vi "4155C Output-FPP Config SMUs v3.0.vi"(0 "VISA resource name in":refnum<visa-resource-name>, 1 "Pulse period":dbl=0.005 min=0.005 max=1.0 step=0.0001 format="%.4f", 2 "FPP - Source":u32(ring)=6 items=["SMU1  ", "SMU2  ", "SMU3  ", "SMU4  ", "SMU5  ", "SMU6  ", "VSU1  ", "VSU2  "], 3 "Pulse width":dbl=0.0005 min=0.0005 max=0.1 step=0.0001 format="%.4f", 4 "Base voltage":dbl format="%^.4e", 5 "error in (no error)":errorcluster, 6 "sweep method":u16(ring) items=["Continuous", "Pulsed"], 7 "FPP - Gate":u32(ring)=2 items=["SMU1  ", "SMU2  ", "SMU3  ", "SMU4  ", "SMU5  ", "SMU6  ", "VSU1  ", "VSU2  "], 8 "FPP - Drain":u32(ring)=1 items=["SMU1  ", "SMU2  ", "SMU3  ", "SMU4  ", "SMU5  ", "SMU6  ", "VSU1  ", "VSU2  "], 9 "FPP - Probe 1":u32(ring) items=["SMU1  ", "SMU2  ", "SMU3  ", "SMU4  ", "SMU5  ", "SMU6  ", "VSU1  ", "VSU2  "], 10 "Gate mode":u16(ring) items=["Auto", "Limited", "Fixed"], 11 "Source/drain mode":u16(ring) items=["Auto", "Limited", "Fixed"], 12 "Gate Range":u8(slide)=6 max=11 scale=0.0..11.0, 13 "Source/drain Range":u8(slide)=6 max=11 scale=0.0..11.0, 15 "FPP - Probe 2":u32(ring)=3 items=["SMU1  ", "SMU2  ", "SMU3  ", "SMU4  ", "SMU5  ", "SMU6  ", "VSU1  ", "VSU2  "]) -> (14 "VISA Resource Name out":refnum<visa-resource-name>, 19 "error out":errorcluster)   [LabVIEW 2016]
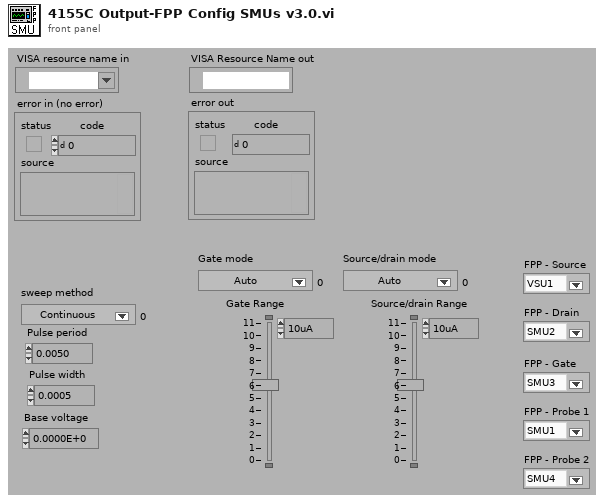
[diagram p1: front panel]
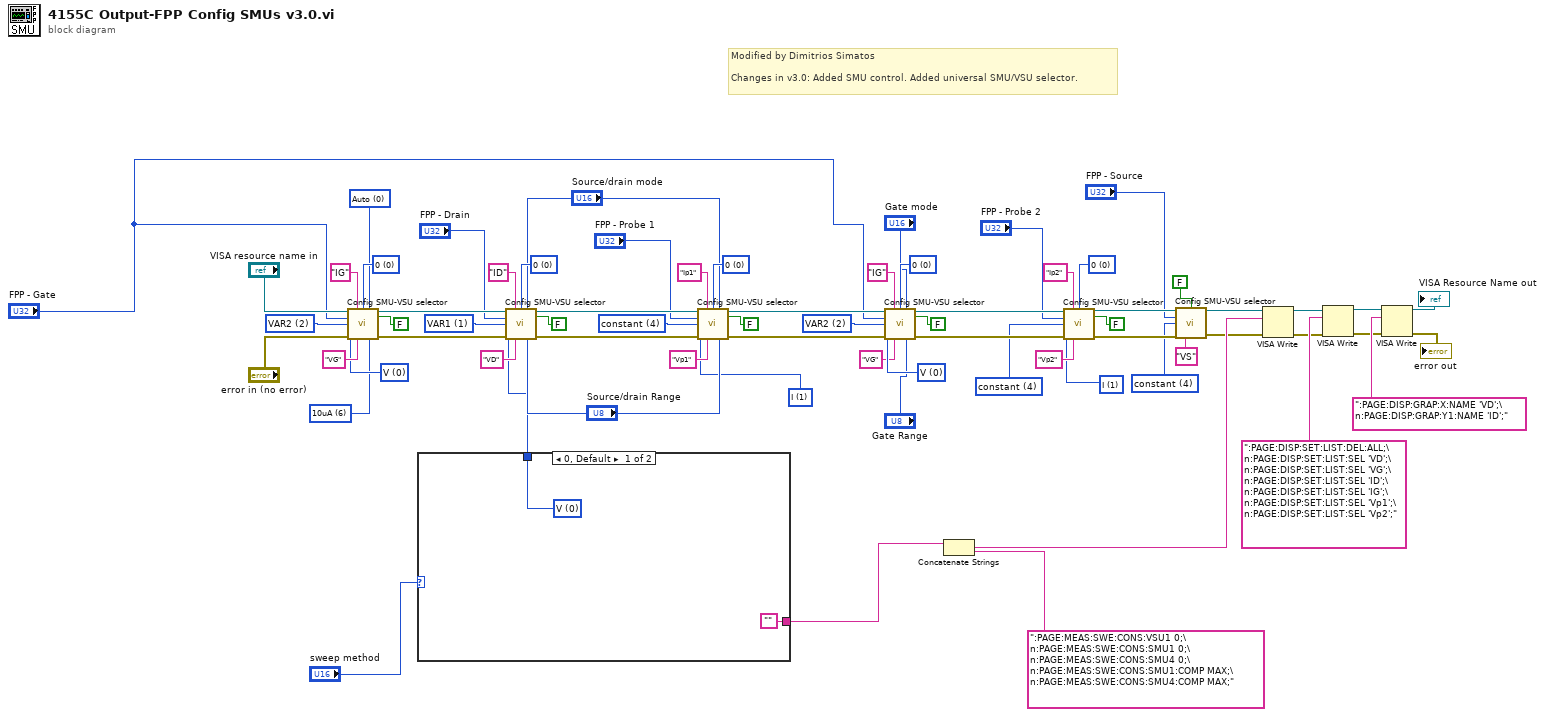
[diagram p0: block diagram]
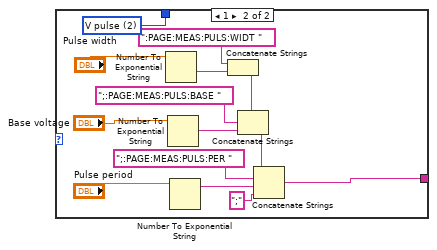
[diagram p2: hidden frame]
diagram:
  w19 = u32 4 items=["disabled  ", "VAR1  ", "VAR2  ", "VAR1'  ", "constant  "] ("function")
  w23 = u32 4 items=["disabled  ", "VAR1  ", "VAR2  ", "VAR1'  ", "constant  "] ("function")
  w25 = u32 1 items=["V  ", "I  ", "V pulse  ", "I pulse  ", "  common  "] ("mode")
  w26 = u16 0 items=["Auto", "Limited", "Fixed"] ("Range mode")
  w27 = u8 6 items=["10fA  ", "100fA  ", "1nA  ", "10nA", "100nA", "1uA", "10uA", "100uA", "1mA", "10mA", "100mA", "1A"] ("Range")
  w32 = u32 2 items=["disabled  ", "VAR1  ", "VAR2  ", "VAR1'  ", "constant  "] ("function")
  w34 = u32 0 items=["0  ", "10K Ohms  ", "100K Ohms  ", "1M Ohms  "] ("series resistance *")
  w35 = u32 0 items=["V  ", "I  ", "V pulse  ", "I pulse  ", "  common  "] ("mode")
  w53 = u32 0 items=["0  ", "10K Ohms  ", "100K Ohms  ", "1M Ohms  "] ("series resistance *")
  w57 = u32 0 items=["V  ", "I  ", "V pulse  ", "I pulse  ", "  common  "] ("mode")
  w58 = u32 0 items=["0  ", "10K Ohms  ", "100K Ohms  ", "1M Ohms  "] ("series resistance *")
  w60 = u32 2 items=["disabled  ", "VAR1  ", "VAR2  ", "VAR1'  ", "constant  "] ("function")
  w63 = u32 0 items=["0  ", "10K Ohms  ", "100K Ohms  ", "1M Ohms  "] ("series resistance *")
  w65 = u32 4 items=["disabled  ", "VAR1  ", "VAR2  ", "VAR1'  ", "constant  "] ("function")
  w39 = u32 1 items=["V  ", "I  ", "V pulse  ", "I pulse  ", "  common  "] ("mode")
  w68 = u32 0 items=["0  ", "10K Ohms  ", "100K Ohms  ", "1M Ohms  "] ("series resistance *")
  w70 = u32 1 items=["disabled  ", "VAR1  ", "VAR2  ", "VAR1'  ", "constant  "] ("function")
  # "Modified by Dimitrios Simatos\n\nChanges in v3.0: Added SMU control. Added universal SMU/VSU selector."
  n1 = call "Config SMU-VSU selector.vi"("VISA session"="VISA resource name in", "I name (max 6 chars)"="IG", "standby"=FALSE, "Range mode"=w26, "unit to configure"="FPP - Gate", "function"=w32, "mode"=w35, "error in (no error)"="error in (no error)", "V name (max 6 chars)"="VG", "series resistance *"=w34, "Range"=w27) -> ("dup VISA resource name"=w29:refnum<visa-resource-name>, "error out"=w30:errorcluster)  [unwired: 1 in, 2 out]
  n2 = case shown="0, Default" "sweep method" {
    tunnel: [w72 w86] -> w38
    tunnel: ["" w77] -> w24
    frame 0, Default {
      w72 = u32 0 items=["V  ", "I  ", "V pulse  ", "I pulse  ", "  common  "] ("mode")
    }
    frame 1 {
      w86 = u32 2 items=["V  ", "I  ", "V pulse  ", "I pulse  ", "  common  "] ("mode")
      n3 = Number To Exponential String(number="Pulse width") -> (E-format string=w85:string)  [unwired: 3 in]
      n4 = Number To Exponential String(number="Base voltage") -> (E-format string=w81:string)  [unwired: 3 in]
      n5 = Number To Exponential String(number="Pulse period") -> (E-format string=w78:string)  [unwired: 3 in]
      n6 = Concatenate Strings(":PAGE:MEAS:PULS:WIDT " ("Substring"), w85) -> (w83:string)
      n7 = Concatenate Strings(w83, ";:PAGE:MEAS:PULS:BASE " ("Substring"), w81) -> (w79:string)
      n8 = Concatenate Strings(w79, ";:PAGE:MEAS:PULS:PER " ("Substring"), w78, ";" ("Substring")) -> (w77:string)
    }
  }
  n9 = call "Config SMU-VSU selector.vi"("VISA session"=w29, "I name (max 6 chars)"="ID", "standby"=FALSE, "Range mode"="Source/drain mode", "unit to configure"="FPP - Drain", "function"=w70, "mode"=w38, "error in (no error)"=w30, "V name (max 6 chars)"="VD", "series resistance *"=w68, "Range"="Source/drain Range") -> ("dup VISA resource name"=w50:refnum<visa-resource-name>, "error out"=w49:errorcluster)  [unwired: 1 in, 2 out]
  n10 = call "Config SMU-VSU selector.vi"("VISA session"=w50, "I name (max 6 chars)"="Ip1", "standby"=FALSE, "Range mode"="Source/drain mode", "unit to configure"="FPP - Probe 1", "function"=w65, "mode"=w39, "error in (no error)"=w49, "V name (max 6 chars)"="Vp1", "series resistance *"=w63, "Range"="Source/drain Range") -> ("dup VISA resource name"=w47:refnum<visa-resource-name>, "error out"=w48:errorcluster)  [unwired: 1 in, 2 out]
  n11 = call "Config SMU-VSU selector.vi"("VISA session"=w47, "I name (max 6 chars)"="IG", "standby"=FALSE, "Range mode"="Gate mode", "unit to configure"="FPP - Gate", "function"=w60, "mode"=w57, "error in (no error)"=w48, "V name (max 6 chars)"="VG", "series resistance *"=w58, "Range"="Gate Range") -> ("dup VISA resource name"=w46:refnum<visa-resource-name>, "error out"=w45:errorcluster)  [unwired: 1 in, 2 out]
  n12 = Concatenate Strings(w24, ":PAGE:MEAS:SWE:CONS:VSU1 0;\n:PAGE:MEAS:SWE:CONS:SMU1 0;\n:PAGE:MEAS:SWE:CONS:SMU4 0;\n:PAGE:MEAS:SWE:CONS:SMU1:COMP MAX;\n:PAGE:MEAS:SWE:CONS:SMU4:COMP MAX;" ("write buffer (\"\")")) -> (w16:string)
  n13 = call "Config SMU-VSU selector.vi"("VISA session"=w46, "I name (max 6 chars)"="Ip2", "standby"=FALSE, "unit to configure"="FPP - Probe 2", "function"=w23, "mode"=w25, "error in (no error)"=w45, "V name (max 6 chars)"="Vp2", "series resistance *"=w53) -> ("dup VISA resource name"=w21:refnum<visa-resource-name>, "error out"=w22:errorcluster)  [unwired: 3 in, 2 out]
  n14 = call "Config SMU-VSU selector.vi"("VISA session"=w21, "standby"=FALSE, "unit to configure"="FPP - Source", "function"=w19, "error in (no error)"=w22, "V name (max 6 chars)"="VS") -> ("dup VISA resource name"=w12:refnum<visa-resource-name>, "error out"=w7:errorcluster)  [unwired: 6 in, 2 out]
  n15 = VISA Write(VISA resource name=w12, write buffer=w16, error in (no error)=w7) -> (VISA resource name out=w17:refnum<visa-resource-name>, error out=w6:errorcluster)  [unwired: 1 out]
  n16 = VISA Write(VISA resource name=w17, write buffer=":PAGE:DISP:SET:LIST:DEL:ALL;\n:PAGE:DISP:SET:LIST:SEL 'VD';\n:PAGE:DISP:SET:LIST:SEL 'VG';\n:PAGE:DISP:SET:LIST:SEL 'ID';\n:PAGE:DISP:SET:LIST:SEL 'IG';\n:PAGE:DISP:SET:LIST:SEL 'Vp1';\n:PAGE:DISP:SET:LIST:SEL 'Vp2';" ("write buffer (\"\")"), error in (no error)=w6) -> (VISA resource name out=w11:refnum<visa-resource-name>, error out=w8:errorcluster)  [unwired: 1 out]
  n17 = VISA Write(VISA resource name=w11, write buffer=":PAGE:DISP:GRAP:X:NAME 'VD';\n:PAGE:DISP:GRAP:Y1:NAME 'ID';" ("write buffer (\"\")"), error in (no error)=w8) -> (VISA resource name out=→"VISA Resource Name out":refnum<visa-resource-name>, error out=→"error out":errorcluster)  [unwired: 1 out]
